vi "getImage.vi"(0 "HGF_IMAQDevice":refnum<class "HGF_IMAQDevice.lvclass">, 2 "Image In":T1, 3 "Buffer Number":u32, 4 "Timeout (1000ms)":i32=1000, 5 "error in (no error)":errorcluster, 6 "Region of Interest":i32[](array[numeric]), 8 "Buffer Number Mode (Next)":T2) -> (11 "Frame Numbers":i32[](array[numeric]), 13 "Image Array":T1[](array[typedef]), 14 "dup HGF_IMAQDevice":refnum<class "HGF_IMAQDevice.lvclass">, 16 "Image Out":T1, 17 "Buffer Number Copied":i32, 18 "Buffer Index Copied":i32, 19 "error out":errorcluster)   [LabVIEW 2014, in "HGF_IMAQ.lvlib" / "HGF_IMAQDevice.lvclass"]
doc: "Returns a copy of an acquired image. IMAQ Copy Acquired Buffer allows you to copy an image from onboard memory to system memory, or from driver-allocated system memory to user-allocated system memory.\n\nCall this VI only after calling IMAQdx Configure Acquisition.vi. If the image type does not match the video format of the camera, this VI changes the image type to a suitable format, at least for IMAQdx."
uses:
  HGF_IMAQDevice.lvclass
  <vilib>/vision/Image Controls.llb/IMAQ Image.ctl
  <vilib>/vision/driver/IMAQdx.llb/IMAQdx Buffer Number Mode.ctl
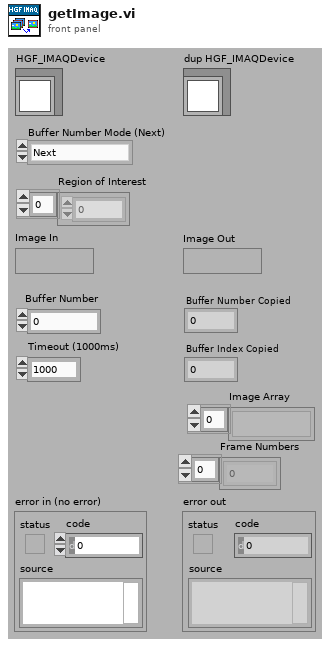
[diagram p1: front panel]
types:
  T1 = typedef "IMAQ Image.ctl" = refnum<image>
  T2 = typedef "NI_Vision_Acquisition_Software.lvlib/IMAQdx Buffer Number Mode.ctl" = enum32{"Next", "Last", "Buffer Number"}
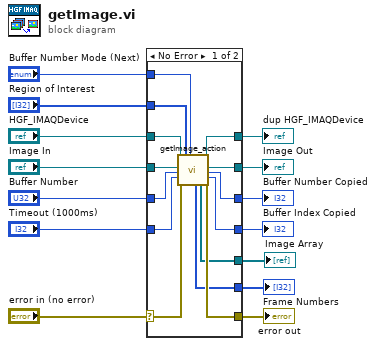
[diagram p0: block diagram]
diagram:
  n1 = case shown="No Error" "error in (no error)" {
    selector: "error in (no error)" -> [w26 w31]
    tunnel: [w25 w31] -> w13
    tunnel: [w27 w30] -> w11
    tunnel: "HGF_IMAQDevice" -> [w28 w30]
    tunnel: "Region of Interest" -> [w24 _]
    tunnel: "Buffer Number Mode (Next)" -> [w23 _]
    tunnel: "Image In" -> [w22 w29]
    tunnel: [w21 w29] -> w7
    tunnel: "Buffer Number" -> [w20 _]
    tunnel: "Timeout (1000ms)" -> [w19 _]
    tunnel: [w18 _] -> w4
    tunnel: [w17 _] -> w3
    tunnel: [w16 _] -> w2
    tunnel: [w15 _] -> w1
    frame No Error {
      n2 = call-dynamic "getImage_action.vi"("HGF_IMAQDevice"=w28, "Image In"=w22, "Buffer Number"=w20, "Timeout (1000ms)"=w19, "error in (no error)"=w26, "Region of Interest"=w24, "Buffer Number Mode (Next)"=w23) -> ("Frame Numbers"=w18:i32[], "Image Array"=w17:T1[], "dup HGF_IMAQDevice"=w27:refnum<class "HGF_IMAQDevice.lvclass">, "Image Out"=w21:T1, "Buffer Number Copied"=w16:i32, "Buffer Index Copied"=w15:i32, "error out"=w25:errorcluster)  [unwired: 6 in]
    }
    frame Error {
    }
  }
  "error out" <- w13
  "dup HGF_IMAQDevice" <- w11
  "Image Array" <- w3
  "Buffer Number Copied" <- w2
  "Buffer Index Copied" <- w1
  "Frame Numbers" <- w4
  "Image Out" <- w7
